vi "LoadRuntimeConf.vi"(11 "Path":path) -> ()   [LabVIEW 2012]
uses:
  <vilib>/Utility/config.llb/Read Key (Double).vi
  <vilib>/Utility/config.llb/NI_LVConfig.lvlib
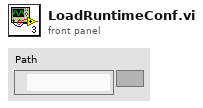
[diagram p1: front panel]
types:
  T1 = typedef "NI_LVConfig.lvlib/Config Data RefNum.ctl" = refnum<k1>
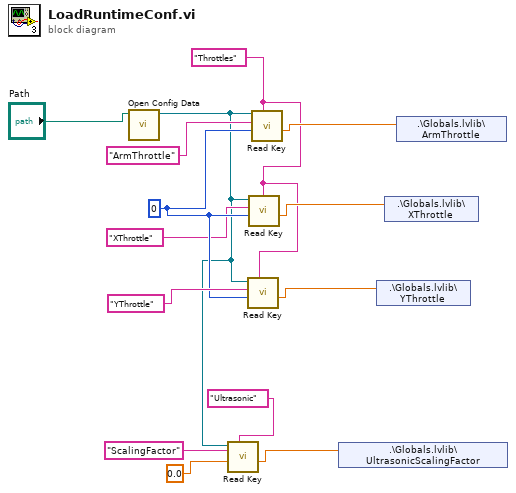
[diagram p0: block diagram]
diagram:
  w9 = 0
  w6 = "Throttles"
  n1 = call <vilib>:"Open Config Data.vi"("configuration file path"="Path") -> ("refnum"=w4:T1)  [unwired: 8 in, 2 out]
  n2 = call-poly <vilib>:"Read Key.vi"("section"="Ultrasonic", "default value"=0.0, "key"="ScalingFactor", "refnum"=w4) -> ("value"=w1:dbl)  [unwired: 4 in, 3 out]
  n3 = call-poly <vilib>:"Read Key.vi"("section"=w6, "default value"=w9, "key"="YThrottle", "refnum"=w4) -> ("value"=w11:dbl)  [unwired: 4 in, 3 out]
  n4 = call-poly <vilib>:"Read Key.vi"("section"=w6, "default value"=w9, "key"="XThrottle", "refnum"=w4) -> ("value"=w12:dbl)  [unwired: 4 in, 3 out]
  n5 = call-poly <vilib>:"Read Key.vi"("section"=w6, "default value"=w9, "key"="ArmThrottle", "refnum"=w4) -> ("value"=w13:dbl)  [unwired: 4 in, 3 out]
  n6 = shared-variable ".\\Globals.lvlib\\UltrasonicScalingFactor"(w1) -> ()  [unwired: 1 in, 1 out]
  n7 = shared-variable ".\\Globals.lvlib\\YThrottle"(w11) -> ()  [unwired: 1 in, 1 out]
  n8 = shared-variable ".\\Globals.lvlib\\XThrottle"(w12) -> ()  [unwired: 1 in, 1 out]
  n9 = shared-variable ".\\Globals.lvlib\\ArmThrottle"(w13) -> ()  [unwired: 1 in, 1 out]
